vi "Boolean Single ref.vi"(0 "controls":refnum<vi>, 1 "Enum":T1(ring), 5 "Visible":bool, 7 "trans":refnum<vi>, 9 "Disabled":T2(ring), 11 "error in (no error)":errorcluster) -> (4 "trans out":refnum<vi>, 6 "controls out":refnum<vi>, 15 "error out":errorcluster)   [LabVIEW 2022 SP3]
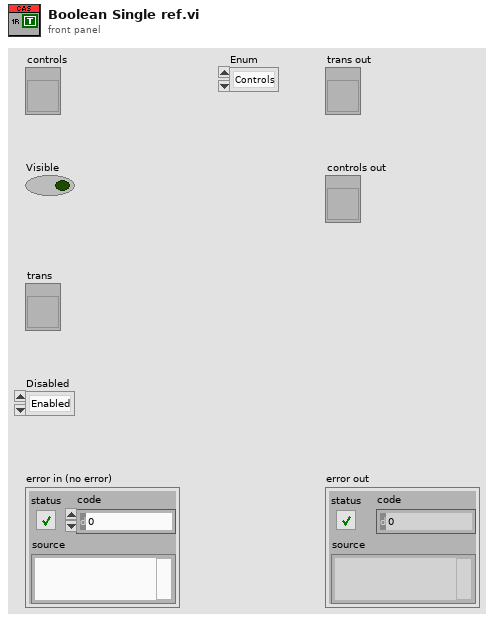
[diagram p1: front panel]
types:
  T1 = enum16{"Controls", "Transparents", "indicators", "Strings"}
  T2 = enum8{"Enabled", "Disabled", "Disabled and Grayed Out"}
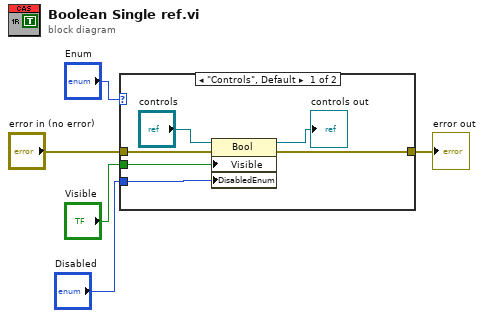
[diagram p0: block diagram]
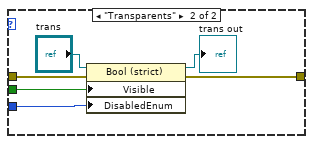
[diagram p2: hidden frame]
diagram:
  n1 = case shown="\"Controls\", Default" "Enum" {
    tunnel: "Visible" -> [w7 w16]
    tunnel: "Disabled" -> [w6 w15]
    tunnel: [w8 w14] -> w3
    tunnel: "error in (no error)" -> [w9 w13]
    frame "Controls", Default {
      n2 = property class="Bool"(reference="controls", error in=w9, "Visible"=w7, "DisabledEnum"=w6) -> (reference out=→"controls out":refnum<vi>, error out=w8:errorcluster)
    }
    frame "Transparents" {
      n3 = property class="Bool (strict)"(reference="trans", error in=w13, "Visible"=w16, "DisabledEnum"=w15) -> (reference out=→"trans out":refnum<vi>, error out=w14:errorcluster)
    }
  }
  "error out" <- w3
